vi "Write Scalar DBL.vi"(8 "error in (no error)":errorcluster, 10 "value":dbl, 11 "pointer in":u64) -> (0 "error out":errorcluster, 2 "value out":dbl, 3 "pointer out":u64)   [LabVIEW 2013, in "Linux RT IPC.Shared Memory.lvlib"]
uses:
  Linux RT IPC.Shared Memory.lvlib
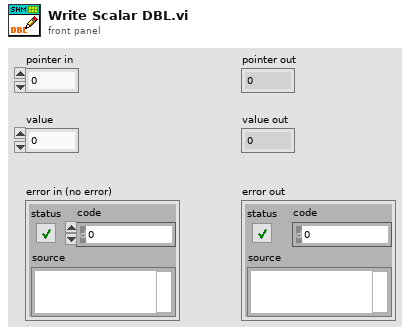
[diagram p1: front panel]
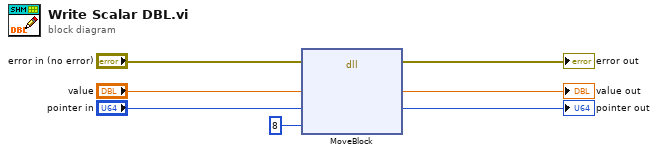
[diagram p0: block diagram]
diagram:
  n1 = dll-call lib="LabVIEW" fn="MoveBlock"(error in="error in (no error)", "data"="value", "pointer"="pointer in", "size"=u64 8) -> (error out=→"error out":errorcluster, "data"=→"value out":dbl, "pointer"=→"pointer out":u64)  [unwired: 4 in, 1 out]
